vi "CRYSingle Limit bar.vi"(11 "Limit Graph":cluster{cluster{"Hz":dbl, dbl}[]}[](array[cluster])) -> (1 "Scale range info":T1 {"Increment" format="%.2f"; "Maximum" format="%.2f"; "Minimum" format="%.2f"}, 2 "Limits bar":cluster{dbl, dbl} {"?" format="%.2f"; "?" format="%.2f"}, 3 "Single value":dbl format="%.2f")   [LabVIEW 2013]
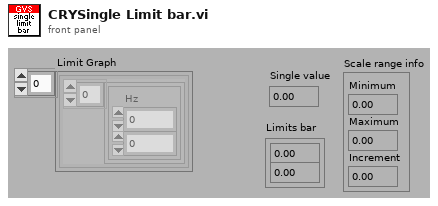
[diagram p1: front panel]
types:
  T1 = cluster{"Minimum":dbl, "Maximum":dbl, "Increment":dbl}
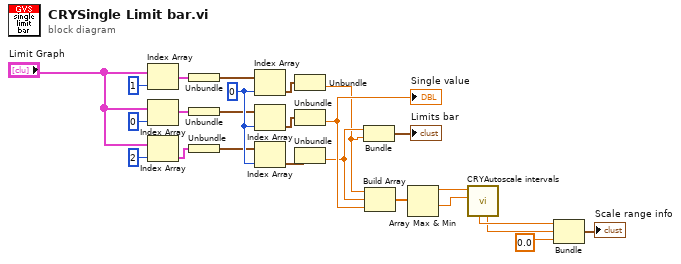
[diagram p0: block diagram]
diagram:
  w19 = 0 ("Index")
  n1 = Index Array(array="Limit Graph", index=1 ("Index")) -> (element=w22:cluster{cluster{"Hz":dbl, dbl}[]})
  n2 = Index Array(array="Limit Graph", index=0 ("Index")) -> (element=w21:cluster{cluster{"Hz":dbl, dbl}[]})
  n3 = Index Array(array="Limit Graph", index=2 ("Index")) -> (element=w20:cluster{cluster{"Hz":dbl, dbl}[]})
  n4 = Unbundle(w22) -> (w18:cluster{"Hz":dbl, dbl}[])
  n5 = Unbundle(w21) -> (w17:cluster{"Hz":dbl, dbl}[])
  n6 = Unbundle(w20) -> (w16:cluster{"Hz":dbl, dbl}[])
  n7 = Index Array(array=w18, index=w19) -> (element=w15:cluster{"Hz":dbl, dbl})
  n8 = Index Array(array=w17, index=w19) -> (element=w14:cluster{"Hz":dbl, dbl})
  n9 = Index Array(array=w16, index=w19) -> (element=w13:cluster{"Hz":dbl, dbl})
  n10 = Unbundle(w15) -> (w1:dbl)  [unwired: 1 out]
  n11 = Unbundle(w14) -> (w11:dbl)  [unwired: 1 out]
  "Single value" <- w11
  n12 = Unbundle(w13) -> (w2:dbl)  [unwired: 1 out]
  n13 = Bundle(w2, w1) -> (→"Limits bar":cluster{dbl, dbl})  [unwired: 1 out]
  n14 = Build Array(w1, w2, w11) -> (w10:dbl[])
  n15 = Array Max & Min(array=w10) -> (max value=w9:dbl, min value=w8:dbl)  [unwired: 2 out]
  n16 = call "CRYAutoscale intervals.vi"("Minimum value (0.0)"=w8, "Maximum value"=w9) -> ("Scale max."=w6:dbl, "Scale min."=w7:dbl)  [unwired: 2 in, 6 out]
  n17 = Bundle("Scale min."=w7, "Scale max."=w6, 0.0) -> (→"Scale range info":cluster{"Scale min.":dbl, "Scale max.":dbl, dbl})  [unwired: 1 out]
